vi "Initialize Analog Module.vi"(7 "Direction":enum16{"Input", "Output"}(ring), 8 "error in (no error)":errorcluster, 9 "FXP Type":string, 10 "Channels":u8, 11 "Module in":refnum<class "Module.lvclass">) -> (0 "error out":errorcluster, 3 "Module out":refnum<class "Module.lvclass">)   [LabVIEW 2015, in "Module.lvclass"]
uses:
  Module.lvclass
  Module Configuration.ctl
  Module.lvclass/Module.ctl
  Loop/Module Loop/Module Loop.lvclass
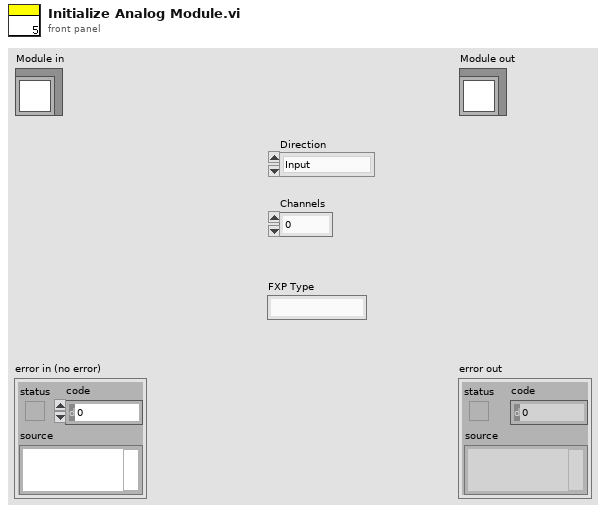
[diagram p1: front panel]
types:
  T1 = typedef "Module Loop.lvclass/Module Configuration.ctl" = cluster{"Type":string, "Direction":string, "Speed":string, "Channels":string, "FXP Type":string}
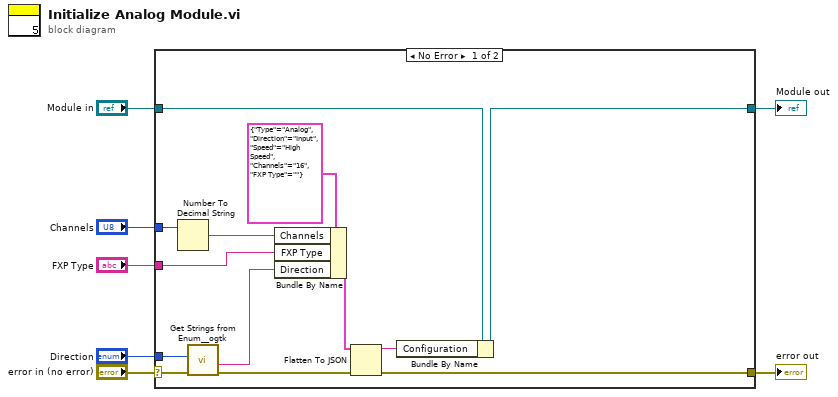
[diagram p0: block diagram]
diagram:
  n1 = case shown="No Error" "error in (no error)" {
    selector: "error in (no error)" -> [w20 w22]
    tunnel: [w12 w22] -> w6
    tunnel: [w8 w21] -> w4
    tunnel: "Module in" -> [w9 w21]
    tunnel: "Direction" -> [w19 _]
    tunnel: "Channels" -> [w16 _]
    tunnel: "FXP Type" -> [w14 _]
    frame No Error {
      n2 = Number To Decimal String(number=w16) -> (decimal integer string=w15:string)  [unwired: 1 in]
      n3 = call <userlib>:"Get Strings from Enum__ogtk.vi"("error in (no error)"=w20, "Enum"=w19) -> ("error out"=w13:errorcluster, "String Value"=w17:string)  [unwired: 6 in, 2 out]
      n4 = Bundle By Name(cluster=T1 {"Type"="Analog", "Direction"="Input", "Speed"="High Speed", "Channels"="16", "FXP Type"=""} ("Cluster"), "Channels"=w15, "FXP Type"=w14, "Direction"=w17) -> (w11:T1)
      n5 = Flatten To JSON(anything=w11, error in (no error)=w13) -> (JSON string=w10:string, 11:w12:errorcluster)  [unwired: 1 in]
      n6 = Bundle By Name(cluster=w9, "Configuration"=w10) -> (w8:refnum<class "Module.lvclass">)
    }
    frame Error {
    }
  }
  "error out" <- w6
  "Module out" <- w4
